vi "test Is Anchor ID Unique False.vi"(8 "error in (no error)":errorcluster, 11 "TestCase in":refnum<class "Utility VIs tests.lvclass">) -> (0 "error out":errorcluster, 3 "TestCase out":refnum<class "Utility VIs tests.lvclass">)   [LabVIEW 2014, in "Utility VIs tests.lvclass"]
uses:
  Utility VIs tests.lvclass
  SPLAT/Anchor/Anchor.lvclass
  <vilib>/addons/_JKI Toolkits/VI Tester/TestCase.llb/TestCase.lvclass
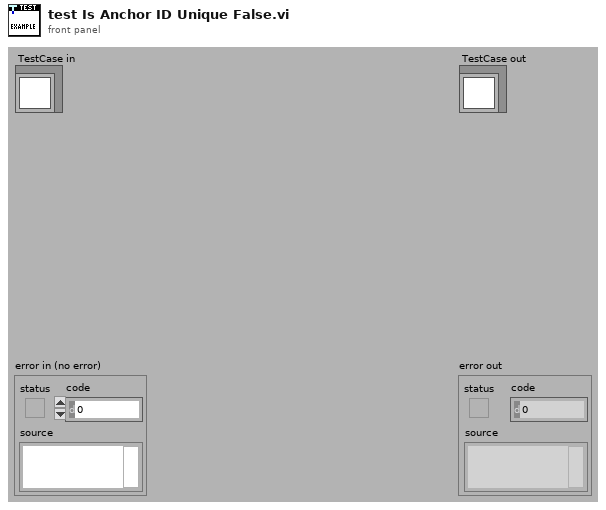
[diagram p1: front panel]
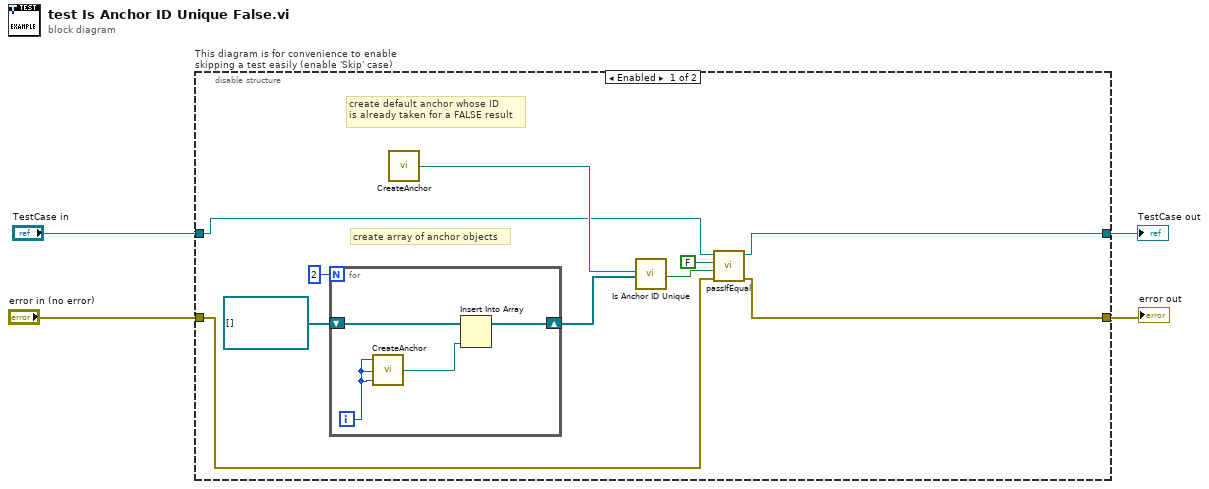
[diagram p0: block diagram]
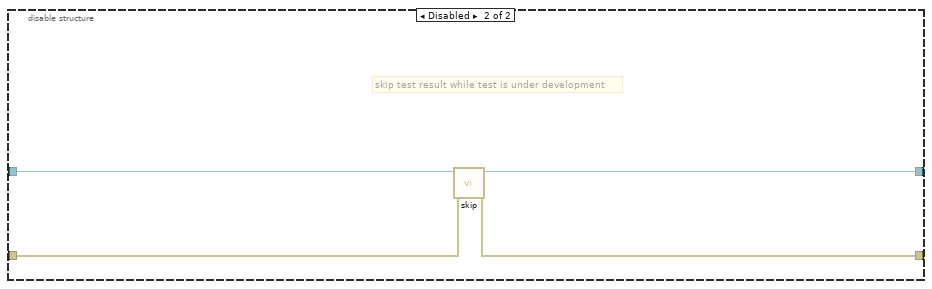
[diagram p2: hidden frame]
diagram:
  n1 = disable-structure "This diagram is for convenience to enable skipping a test easily (enable 'Skip' case)" shown="Enabled" {
    disable-tunnel: "TestCase in" -> [w9 w22]
    disable-tunnel: [w8 w20] -> w1
    disable-tunnel: [w6 w21] -> w3
    disable-tunnel: "error in (no error)" -> [w7 w19]
    frame Enabled {
      # "create default anchor whose ID \nis already taken for a FALSE result"
      # "create array of anchor objects"
      n2 = for {
        N: 2 -> [_]
        shift-right: [w17] -> w13
        shift-left: refnum<class "Anchor.lvclass">[] [] -> [w18]
        i -> [w16]
        n3 = call "CreateAnchor.vi"("Anchor Y"=w16, "Anchor X"=w16, "Anchor ID"=w16) -> ("Anchor Out"=w15:refnum<class "Anchor.lvclass">)
        n4 = Insert Into Array(array=w18, new element=w15) -> (w17:refnum<class "Anchor.lvclass">[])  [unwired: 1 in]
      }
      n5 = call "CreateAnchor.vi"() -> ("Anchor Out"=w12:refnum<class "Anchor.lvclass">)  [unwired: 3 in]
      n6 = call "Is Anchor ID Unique.vi"("Anchor.lvclass"=w12, "Input AnchorArray"=w13) -> ("Is unique?"=w11:bool)  [unwired: 17 in]
      n7 = call-dynamic "passIfEqual.vi"("error in (no error)"=w7, "y"=w11, "x"=FALSE, "TestCase in"=w9) -> ("error out"=w6:errorcluster, "TestCase out"=w8:refnum<class "Utility VIs tests.lvclass">)  [unwired: 6 in]
    }
    frame Disabled {
      # "skip test result while test is under development"
      n8 = call <vilib>:"skip.vi"("error in (no error)"=w19, "TestCase in"=w22) -> ("error out"=w21:errorcluster, "TestCase out"=w20:refnum<class "Utility VIs tests.lvclass">)  [unwired: 8 in]
    }
  }
  "error out" <- w3
  "TestCase out" <- w1
